vi "permutate.vi"(11 "Input":string[](array[string])=["", "", "", "", ""]) -> (3 "permutations":string[][](array[string]))   [LabVIEW 2021]
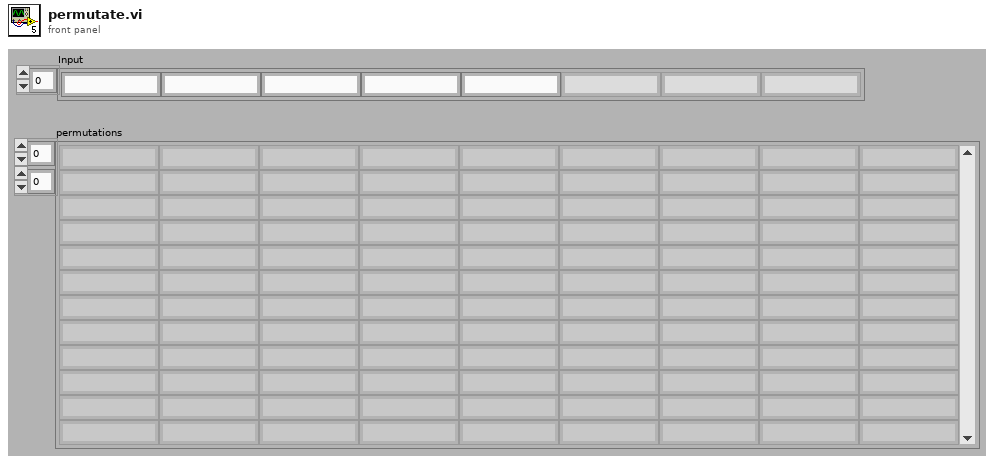
[diagram p1: front panel]
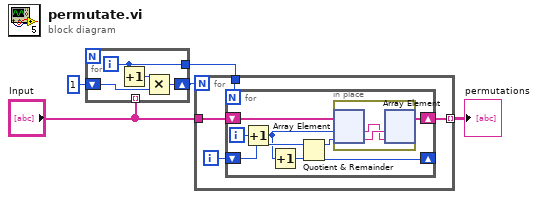
[diagram p0: block diagram]
diagram:
  n1 = for {
    shift-right: [w8] -> w4
    shift-left: 1 -> [w7]
    tunnel: "Input" -> [_] mode=indexing
    tunnel: [w6] -> w2
    i -> [w6]
    n2 = Increment(x=w6) -> (x+1=w9:i32)
    n3 = Multiply(x=w9, y=w7) -> (x*y=w8:i32)
  }
  n4 = for {
    N: w4 -> [_]
    tunnel: w2 -> [w13]
    tunnel: "Input" -> [w12]
    tunnel: [w10] -> w1 mode=indexing
    i -> [w11]
    n5 = for "loop over j (2..length(s))" {
      N: w13 -> [_]
      shift-right: [w14] -> w10
      shift-left: w12 -> [w16]
      shift-right: [w19] -> _
      shift-left: w11 -> [w21]
      i -> [w20]
      n6 = Increment(x=w20) -> (x+1=w17:i32)
      n7 = Increment(x=w17) -> (x+1=w18:i32)
      n8 = Quotient & Remainder(x=w21, y=w18) -> (x-y*floor(x/y)=w15:i32, floor(x/y)=w19:i32)
      n9 = in-place {
        n10 = in-place-array #1(w16, w17, w15) -> (w22:string, w23:string)
        n11 = in-place-array #1(w23, w22) -> (w14:string[])  [unwired: 2 out]
      }
    }
  }
  "permutations" <- w1
